vi "copyConfigFiles.vi"(8 "error in (no error)":errorcluster, 11 "Destination":path) -> (0 "error out":errorcluster)   [LabVIEW 2015]
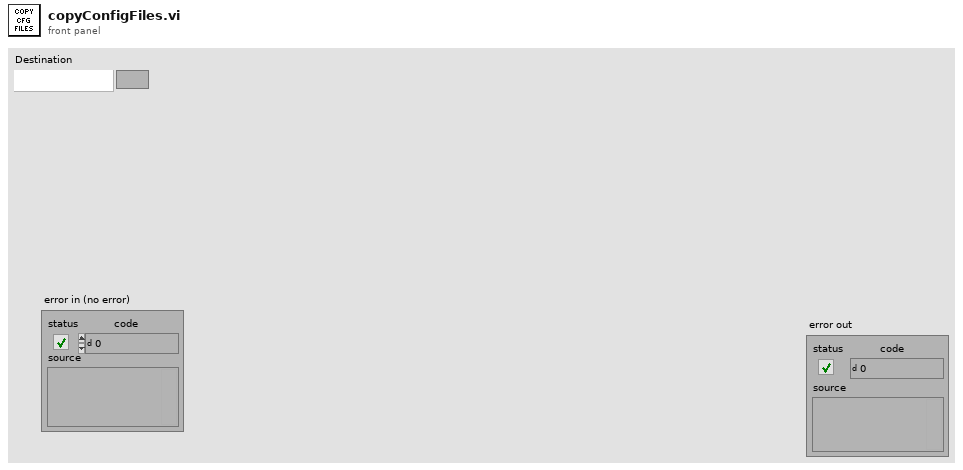
[diagram p1: front panel]
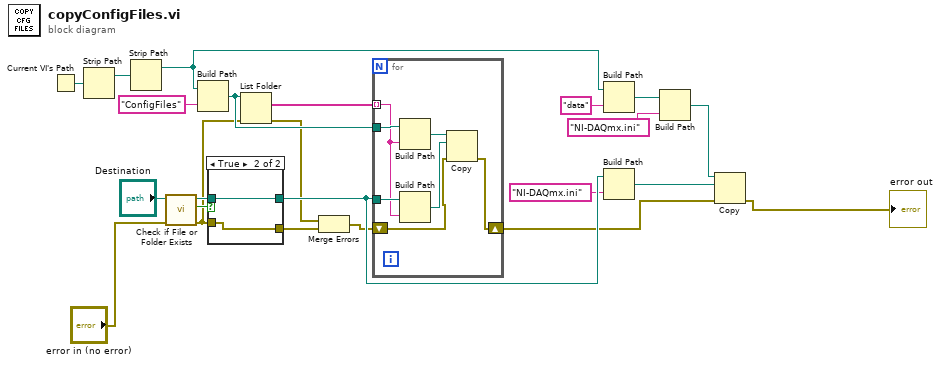
[diagram p0: block diagram]
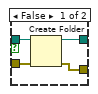
[diagram p2: hidden frame]
diagram:
  n1 = Current VI's Path() -> (path=w10:path)
  n2 = Strip Path(path=w10) -> (stripped path=w2:path)  [unwired: 1 out]
  n3 = Strip Path(path=w2) -> (stripped path=w1:path)  [unwired: 1 out]
  n4 = call <vilib>:"Check if File or Folder Exists.vi"("error in (no error)"="error in (no error)", "path"="Destination") -> ("error out"=w8:errorcluster, "file or folder exists?"=w19:bool, "dup path"=w18:path)  [unwired: 7 in]
  n5 = Build Path(base path=w1, name or relative path="ConfigFiles") -> (appended path=w21:path)
  n6 = case shown="True" w19 {
    tunnel: w18 -> [w27 w29]
    tunnel: [w26 w29] -> w14
    tunnel: w8 -> [w25 w28]
    tunnel: [w24 w28] -> w7
    frame False {
      n7 = Create Folder(path (use dialog)=w27, error in=w25) -> (created path=w26:path, error out=w24:errorcluster)  [unwired: 1 in, 1 out]
    }
    frame True {
    }
  }
  n8 = List Folder(path=w21, error in=w8) -> (filenames=w22:string[], error out=w5:errorcluster)  [unwired: 2 in, 2 out]
  n9 = Merge Errors(w5, w7) -> (w6:errorcluster)
  n10 = for {
    tunnel: w22 -> [w34] mode=indexing
    tunnel: w21 -> [w36]
    tunnel: w14 -> [w35]
    shift-right: [w30] -> w4
    shift-left: w6 -> [w31]
    n11 = Build Path(base path=w36, name or relative path=w34) -> (appended path=w32:path)
    n12 = Build Path(base path=w35, name or relative path=w34) -> (appended path=w33:path)
    n13 = Copy(8:w31, 10:w33, 11:w32) -> (0:w30:errorcluster)  [unwired: 2 in, 2 out]
  }
  n14 = Build Path(base path=w1, name or relative path="data") -> (appended path=w16:path)
  n15 = Build Path(base path=w14, name or relative path="NI-DAQmx.ini") -> (appended path=w11:path)
  n16 = Build Path(base path=w16, name or relative path="NI-DAQmx.ini") -> (appended path=w12:path)
  n17 = Copy(8:w4, 10:w11, 11:w12) -> (0:→"error out":errorcluster)  [unwired: 2 in, 2 out]
